vi "Drive Controller.vi"(8 "error in":errorcluster) -> ()   [LabVIEW 2019]
doc: "This VI executes continuously carrying out the current operation and responding to updates or new operation requests. It will often contain the timing or control code that is difficult to place directly in TeleOp. This VI generally opens all sensors and motors and isolates the rest of the robot code from knowing implementation details of how the operations are carried out."
uses:
  <vilib>/Rock Robotics/WPI/Framework/Completion Status.ctl
  Drive Setpoints.ctl
  Drive Operations.ctl
  <vilib>/Rock Robotics/WPI/SafetyOutput/WPI_SafetyOutputConfigMenu.ctl
  <vilib>/Rock Robotics/WPI/Utilities/WPI_GetSetVariantRefNum.vi
panel:
  in  "Interactive Values":T1
  in  "Buttons":cluster{"Execute Cmd":bool, "Abort Cmd":bool}
  out "Command Timing":cluster{"Start Time (ms)":u32, "Iterations":i32}
  out "Status":T3
  out "Setpoints":T4(graph)
  out "Current\nCmd":string
  # "Tip: The graph shows the motor setpoints. It may also be helpful to observe inputs and sensor values.\nYou may also want to display tuning or debugging controls."
  # "Interactive Command: You may fill in the settings for a command\nand schedule it with the Execute button. You can observe and abort\nany command while fine tuning the code for the controller."
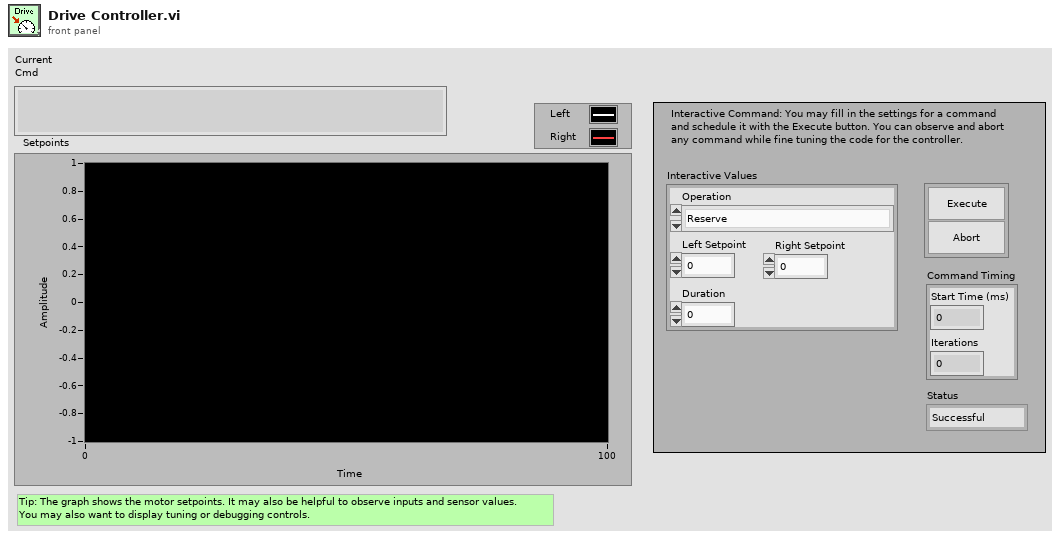
[diagram p1: front panel]
types:
  T1 = typedef "Drive Setpoints.ctl" = cluster{"Operation":T2, "Left Setpoint":dbl, "Right Setpoint":dbl, "Duration":dbl}
  T2 = typedef "Drive Operations.ctl" = enum16{"Reserve", "Read Current", "Immediate", "Drive for Time", "Drive for Distance", "Turn Left", "Turn Right"}
  T3 = typedef "Completion Status.ctl" = enum16{"Successful", "Aborted", "Incomplete"}
  T4 = cluster{"Left Setpoint":dbl, "Right Setpoint":dbl}
  T5 = typedef "WPI_SafetyOutputConfigMenu.ctl" = enum16{"Enable", "Disable"}
  T6 = typedef "WPI_RobotDriveDevRef.ctl" = cluster{"DevStatus":errorcluster, "Motors[]":T7[], "Square Inputs":bool, "Max Output":dbl}
  T7 = typedef "WPI_MotorControlDeviceRef.ctl" = cluster{"DeviceStatus":errorcluster, "Type":T8, "PWM":cluster{"PWM Channel":T9, "DeadBand":T10}, "CAN":cluster{"Device Number":u8, "SetOutput VI Ref":variant, "GetOutput VI Ref":variant, "Enable VI Ref":variant, "Disable VI Ref":variant, "Data":variant}, "Invert":bool, "DIO PWM":cluster{"PWM \"Enable\" Channel":T9, "DIOChannel":T11, "PWM Rate":dbl}}
  T8 = typedef "WPI_MotorControlType.ctl" = enum16{"PWM", "CAN", "DIO PWM"}
  T9 = typedef "FPGA_DIOPWMChannel.ctl" = enum8{"PWM 0", "PWM 1", "PWM 2", "PWM 3", "PWM 4", "PWM 5", "PWM 6", "PWM 7", "PWM 8", "PWM 9", "PWM MXP 0", "PWM MXP 1", "PWM MXP 2", "PWM MXP 3", "PWM MXP 4", "PWM MXP 5", "PWM MXP 6", "PWM MXP 7", "PWM MXP 8", "PWM MXP 9", "Invalid"}
  T10 = typedef "WPI_PWMDeadband.ctl" = cluster{"Name":string, "maxPositivePwm":i32, "minPositivePwm":i32, "centerPwm":i32, "maxNegativePwm":i32, "minNegativePwm":i32, "angularRange":u16}
  T11 = typedef "FPGA_DIOChannel.ctl" = enum8{"DIO 0", "DIO 1", "DIO 2", "DIO 3", "DIO 4", "DIO 5", "DIO 6", "DIO 7", "DIO 8", "DIO 9", "DIO MXP 0", "DIO MXP 1", "DIO MXP 2", "DIO MXP 3", "DIO MXP 4", "DIO MXP 5", "DIO MXP 6", "DIO MXP 7", "DIO MXP 8", "DIO MXP 9", "DIO MXP 10", "DIO MXP 11", "DIO MXP 12", "DIO MXP 13", "DIO MXP 14", "DIO MXP 15", "SPI Port CS1", "SPI Port CS2", "SPI Port CS3", "SPI Port MISO", "SPI Port MOSI", "Invalid"}
  T12 = typedef "Command Status Info.ctl" = cluster{"Name":string, "Status":T3, "notifier out":T13}
  T13 = typedef "Completion Notifier.ctl" = refnum<notifier>
  T14 = cluster{"SubSystem Data":T1, cluster{"Start Time (ms)":u32, "Iterations":i32}, cluster{"Command Info":T12, "Description":string, "Default Command":T1, "queue out":refnum<queue>, "Subsystem Name":string}}
  T15 = cluster{"SubSystem Data":T1, cluster{"Start Time (ms)":u32, "Iterations":i32}, "Default Command Arguments":cluster{"Command Info":T12, "Description":string, "Default Command":T1, "queue out":refnum<queue>, "Subsystem Name":string}}
  T16 = cluster{"Don't move motors while reserved":dbl, "Don't move motors while reserved":dbl}
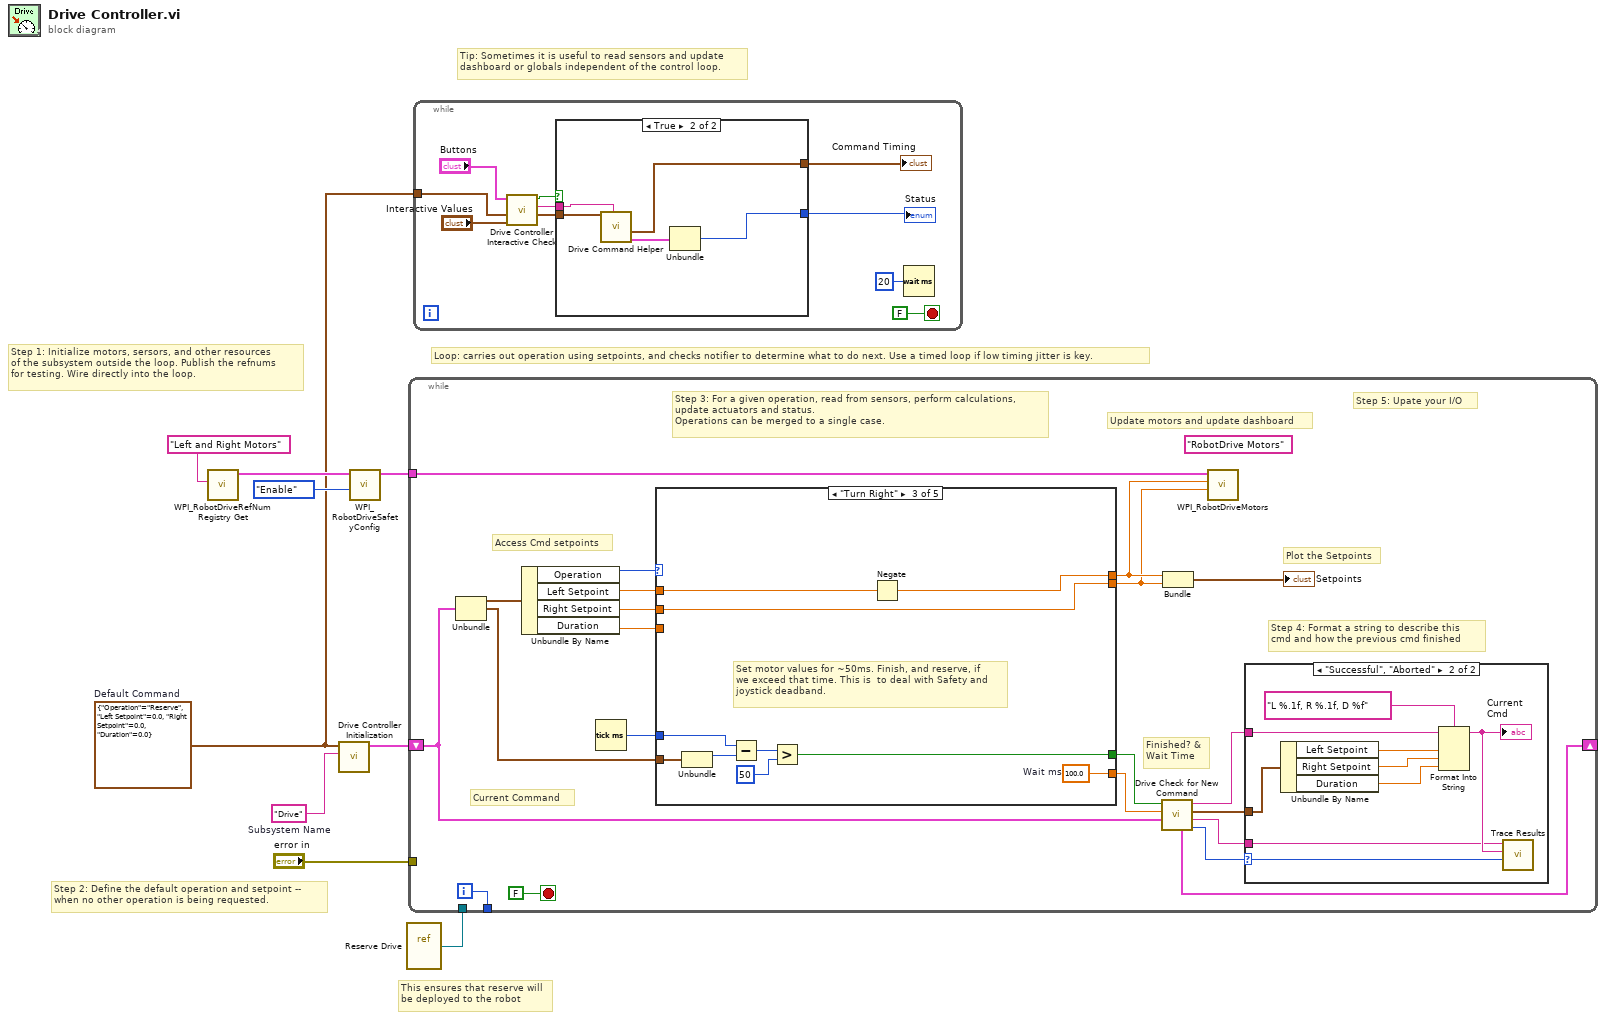
[diagram p0: block diagram]
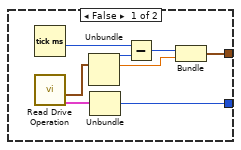
[diagram p2: hidden frame]
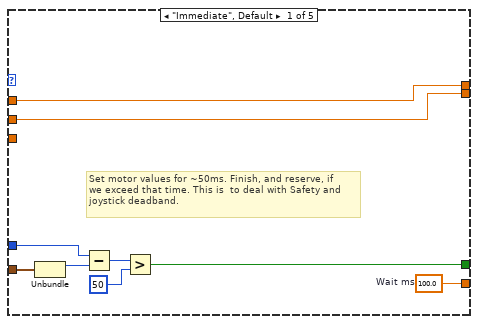
[diagram p4: hidden frame]
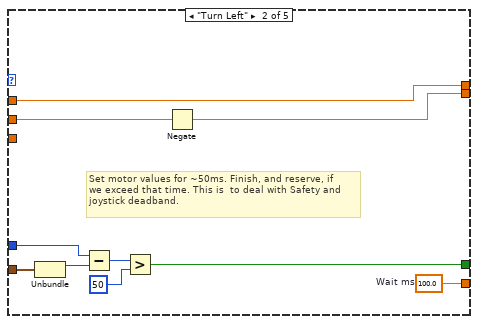
[diagram p5: hidden frame]
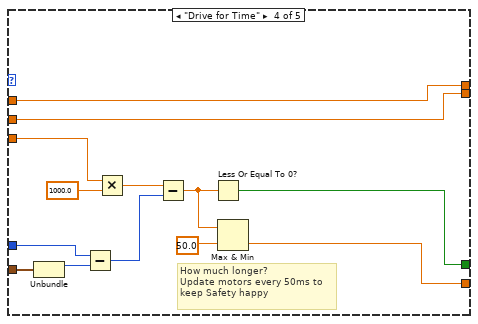
[diagram p6: hidden frame]
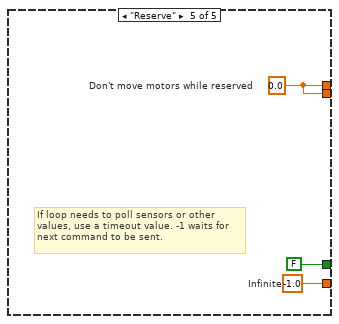
[diagram p7: hidden frame]
diagram:
  w1 = T1 {"Operation"=enum."Reserve", "Left Setpoint"=0.0, "Right Setpoint"=0.0, "Duration"=0.0}  # Default Command
  w9 = "Drive"  # Subsystem Name
  # "This ensures that reserve will\nbe deployed to the robot"
  # "Tip: Sometimes it is useful to read sensors and update\ndashboard or globals independent of the control loop."
  # "Step 2: Define the default operation and setpoint --\nwhen no other operation is being requested."
  # "Step 1: Initialize motors, sersors, and other resources\nof the subsystem outside the loop. Publish the refnums\nfor testing. Wire directly into the loop."
  # "Loop: carries out operation using setpoints, and checks notifier to determine what to do next. Use a timed loop if low timing jitter is key."
  n1 = call <vilib>:"WPI_RobotDriveRefNum Registry Get.vi"("refnum name"="Left and Right Motors") -> ("RobotDriveDevRef"=w7:T6)  [unwired: 9 in, 1 out]
  n2 = call "Drive Controller Initialization.vi"("Subsystem Name"=w9, "Default Command"=w1) -> ("Current Command"=w3:T14)  [unwired: 9 in]
  n3 = call <vilib>:"WPI_RobotDriveSafetyConfig.vi"("mode"=WPI_SafetyOutputConfigMenu."Enable", "RobotDriveDevRef"=w7) -> ("RobotDriveDevRef"=w5:T6)  [unwired: 8 in, 1 out]
  n4 = vi-ref "Reserve Drive.vi"() -> (w2:refnum<vi>)
  n5 = while {
    shift-right: [w17] -> _
    shift-left: w3 -> [w10]
    tunnel: [w29] -> _
    tunnel: w5 -> [w25]
    tunnel: "error in" -> [_]
    tunnel: w2 -> [_]
    i -> [w29]
    stop <- FALSE stop-if-true
    (unwired) "RobotDrive Motors" ("Name")
    # "Step 5: Upate your I/O"
    # "Step 4: Format a string to describe this\ncmd and how the previous cmd finished"
    # "Current Command"
    # "Update motors and update dashboard"
    # "Plot the Setpoints"
    # "Access Cmd setpoints"
    # "Finished? &\nWait Time"
    # "Step 3: For a given operation, read from sensors, perform calculations,\nupdate actuators and status.\nOperations can be merged to a single case."
    n6 = Unbundle(w10) -> ("SubSystem Data"=w24:T1, w11:cluster{"Start Time (ms)":u32, "Iterations":i32})  [unwired: 1 out]
    n7 = Unbundle By Name(w24) -> ("Operation"=w23:T2, "Left Setpoint"=w22:dbl, "Right Setpoint"=w21:dbl, "Duration"=w20:dbl)
    n8 = Tick Count (ms)() -> (millisecond timer value=w19:u32)
    n9 = case shown="\"Turn Right\"" w23 {
      tunnel: [w48 w58 w68 w69 w84] -> w16
      tunnel: [w41 w51 w61 w76 FALSE ("ignore previous (F)")] -> w15
      tunnel: w11 -> [w40 w50 w60 w78 _]
      tunnel: [w47 w57 w59 w75 w82] -> w27
      tunnel: [w46 w49 w66 w74 w82] -> w26
      tunnel: w22 -> [w47 w57 w67 w75 _]
      tunnel: w21 -> [w46 w56 w66 w74 _]
      tunnel: w20 -> [_ _ _ w73 _]
      tunnel: w19 -> [w42 w52 w62 w72 _]
      frame "Immediate", Default {
        w48 = 100.0  # Wait ms
        # "Set motor values for ~50ms. Finish, and reserve, if\nwe exceed that time. This is  to deal with Safety and\njoystick deadband."
        n10 = Unbundle(w40) -> ("Start Time (ms)"=w43:u32)  [unwired: 1 out]
        n11 = Subtract(x=w42, y=w43) -> (x-y=w44:u32)
        n12 = Greater?(x=w44, y=u8 50 ("Left Motor")) -> (0:w41:bool)
      }
      frame "Turn Left" {
        w58 = 100.0  # Wait ms
        # "Set motor values for ~50ms. Finish, and reserve, if\nwe exceed that time. This is  to deal with Safety and\njoystick deadband."
        n13 = Unbundle(w50) -> ("Start Time (ms)"=w53:u32)  [unwired: 1 out]
        n14 = Subtract(x=w52, y=w53) -> (x-y=w54:u32)
        n15 = Greater?(x=w54, y=u8 50 ("Left Motor")) -> (0:w51:bool)
        n16 = Negate(x=w56) -> (-x=w49:dbl)
      }
      frame "Turn Right" {
        w68 = 100.0  # Wait ms
        # "Set motor values for ~50ms. Finish, and reserve, if\nwe exceed that time. This is  to deal with Safety and\njoystick deadband."
        n17 = Unbundle(w60) -> ("Start Time (ms)"=w63:u32)  [unwired: 1 out]
        n18 = Subtract(x=w62, y=w63) -> (x-y=w64:u32)
        n19 = Greater?(x=w64, y=u8 50 ("Left Motor")) -> (0:w61:bool)
        n20 = Negate(x=w67) -> (-x=w59:dbl)
      }
      frame "Drive for Time" {
        # "How much longer?\nUpdate motors every 50ms to\nkeep Safety happy"
        n21 = Unbundle(w78) -> ("Start Time (ms)"=w77:u32)  [unwired: 1 out]
        n22 = Subtract(x=w72, y=w77) -> (x-y=w81:u32)
        n23 = Multiply(x=w73, y=1000.0) -> (x*y=w80:dbl)
        n24 = Subtract(x=w80, y=w81) -> (x-y=w71:dbl)
        n25 = Less Or Equal To 0?(x=w71) -> (x <= 0?=w76:bool)
        n26 = Max & Min(x=w71, y=50.0) -> (min(x,y)=w69:dbl)  [unwired: 1 out]
      }
      frame "Reserve" {
        w82 = 0.0  # Don't move motors while reserved
        w84 = -1.0  # Infinite
        # "If loop needs to poll sensors or other\nvalues, use a timeout value. -1 waits for\nnext command to be sent."
      }
    }
    n27 = call "Drive Check for New Command.vi"("input cluster"=w10, "Wait time (ms)"=w16, "Finished?"=w15) -> ("Completion"=w18:T3, "Subsystem Name"=w12:string, "Current Command"=w13:T1, "Initial Trace String"=w14:string, "Next Command"=w17:T15)  [unwired: 4 in]
    n28 = Bundle("Don't move motors while reserved"=w27, "Don't move motors while reserved"=w26) -> (→"Setpoints":T16)  [unwired: 1 in]
    n29 = call <vilib>:"WPI_RobotDriveMotors.vi"("RightSpeed"=w26, "LeftSpeed"=w27, "RobotDriveDevRef"=w25) -> ()  [unwired: 1 in, 8 out]
    n30 = case shown="\"Successful\", \"Aborted\"" w18 {
      selector: w18 -> [_ w39]
      tunnel: w14 -> [_ w34]
      tunnel: w13 -> [_ w35]
      tunnel: w12 -> [_ w31]
      frame "Incomplete", Default {
        # "Continuing current command"
      }
      frame "Successful", "Aborted" {
        # "Report and setup for next command"
        n31 = Unbundle By Name(w35) -> ("Left Setpoint"=w37:dbl, "Right Setpoint"=w38:dbl, "Duration"=w32:dbl)
        n32 = Format Into String(format string="L %.1f, R %.1f, D %f", initial string=w34, w37, w38, w32) -> (resulting string=w33:string)  [unwired: 1 in, 1 out]
        "Current\nCmd" <- w33
        n33 = call <vilib>:"Trace Results.vi"("Status of previous command"=w39, "Description"=w33, "Subsystem"=w31) -> ()  [unwired: 9 in]
      }
    }
  }
  n34 = while {
    tunnel: w1 -> [w86]
    stop <- FALSE stop-if-true
    n35 = call "Drive Controller Interactive Check.vi"("Interactive Command In"="Interactive Values", "Default Command"=w86, "Buttons"="Buttons") -> ("Interactive Command Out"=w88:T1, "Trace String"=w89:string, "Schedule"=w90:bool)  [unwired: 6 in]
    n36 = case shown="True" w90 {
      tunnel: [w99 w107] -> w91
      tunnel: [w98 w103] -> w92
      tunnel: w89 -> [_ w105]
      tunnel: w88 -> [_ w104]
      frame False {
        n37 = Tick Count (ms)() -> (millisecond timer value=w102:u32)
        n38 = call "Read Drive Operation.vi"() -> ("Command Info"=w96:T12, "SubSystem Data"=w95:T1)  [unwired: 9 in, 1 out]
        n39 = Unbundle(w95) -> ("Operation"=w100:T2, "Left Setpoint"=w97:dbl)  [unwired: 2 out]
        n40 = Unbundle(w96) -> ("Status"=w99:T3)  [unwired: 2 out]
        n41 = Subtract(x=w102, y=w100) -> (x-y=w101:u32)
        n42 = Bundle(w101, "Left Setpoint"=w97) -> (w98:cluster{u32, "Left Setpoint":dbl})  [unwired: 1 in]
      }
      frame True {
        n43 = call "Drive Command Helper.vi"("Description"=w105, "SubSystem Data"=w104) -> ("Command Info Out"=w106:T12, "Command Timing"=w103:cluster{"Start Time (ms)":u32, "Iterations":i32})  [unwired: 7 in, 1 out]
        n44 = Unbundle(w106) -> ("Status"=w107:T3)  [unwired: 2 out]
      }
    }
    "Status" <- w91
    "Command Timing" <- w92
    n45 = Wait (ms)(milliseconds to wait=u32 20) -> ()  [unwired: 1 out]
  }
